vi "Get Wizard Config Path.vi"(8 "error in (no error)":errorcluster) -> (0 "error out":errorcluster, 2 "Wizard Config Path":path, 3 "Config File Exists":bool)   [LabVIEW 2018]
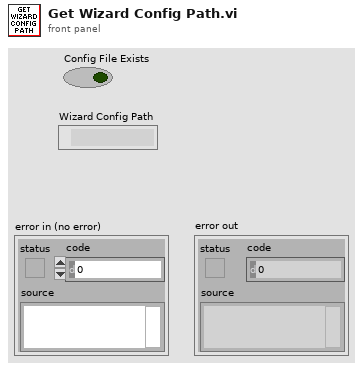
[diagram p1: front panel]
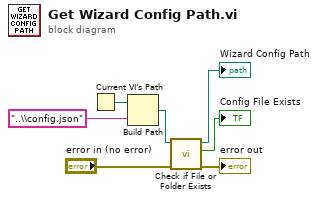
[diagram p0: block diagram]
diagram:
  n1 = Current VI's Path() -> (path=w3:path)
  n2 = Build Path(base path=w3, name or relative path="..\\config.json") -> (appended path=w5:path)
  n3 = call <vilib>:"Check if File or Folder Exists.vi"("error in (no error)"="error in (no error)", "path"=w5) -> ("error out"=→"error out":errorcluster, "file or folder exists?"=→"Config File Exists":bool, "dup path"=→"Wizard Config Path":path)  [unwired: 7 in]
